vi "Encode JSON.vi"(4 "error in (no error)":errorcluster, 7 "JSON Tree":variant) -> (0 "error out":errorcluster, 2 "String":string)   [LabVIEW 2011, in "i3-json.lvlib"]
uses:
  i3-json.lvlib
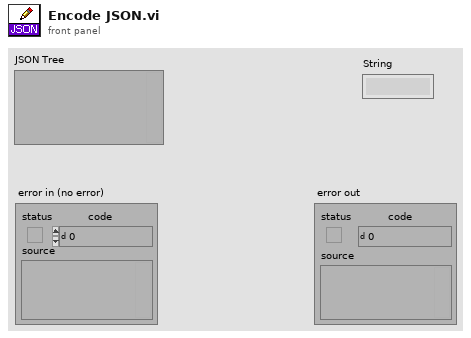
[diagram p1: front panel]
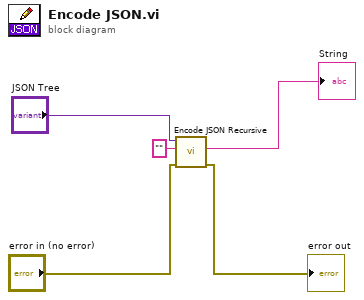
[diagram p0: block diagram]
diagram:
  n1 = call "Encode JSON Recursive.vi"("error in (no error)"="error in (no error)", "String In"="", "JSON Tree"="JSON Tree") -> ("error out"=→"error out":errorcluster, "String Out"=→"String":string)  [unwired: 3 in]
